vi "Close.vi"   [LabVIEW 2021, in "Field_RnD_Services_LIBSSH2_Toolkit.lvlib" / "SFTP Directory.lvclass"]
doc: "Deallocates, or frees, the memory allocated for the libssh2lv shared library SFTP Directory struct represented by this SFTP Directory object. After this is called, the object can no longer be used in the application without causing a segmentation fault, i.e. crashing LabVIEW. This VI must be called to avoid leaking memory or running Out-of-Memory (OOM) on resource-constrained systems."
uses:
  SFTP Directory.lvclass
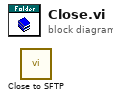
[diagram p0: block diagram]
diagram:
  n1 = call "Close to SFTP.vi"() -> ()  [unwired: 9 in, 3 out]
